vi "Create Result File Name.vi"(6 "Extension":string, 8 "error in (no error)":errorcluster, 9 "File No.":i32 min=0 max=9999 step=1, 10 "Prefix":string="US", 11 "Result Directory":path) -> (0 "error out":errorcluster, 1 "File Name":string, 3 "Result File Path":path)   [LabVIEW 2016]
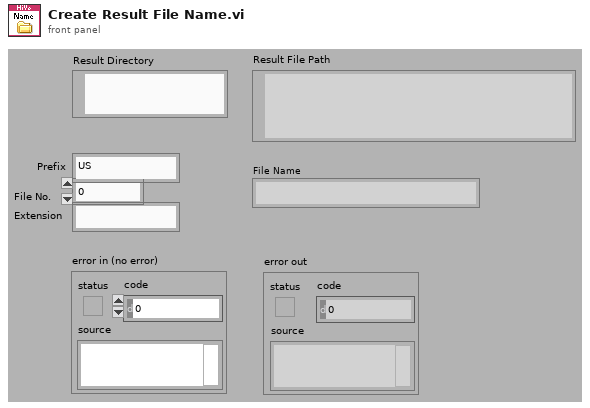
[diagram p1: front panel]
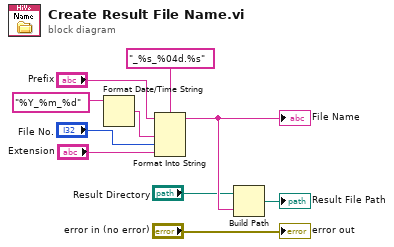
[diagram p0: block diagram]
diagram:
  n1 = Format Date/Time String(time format string (%c)="%Y_%m_%d") -> (date/time string=w6:string)  [unwired: 2 in]
  n2 = Format Into String(format string="_%s_%04d.%s", initial string="Prefix", w6, "File No.", "Extension") -> (resulting string=w9:string)  [unwired: 1 in, 1 out]
  "File Name" <- w9
  n3 = Build Path(base path="Result Directory", name or relative path=w9) -> (appended path=→"Result File Path":path)
  "error out" <- "error in (no error)"
